vi "Teleop_Calc_Forward.vi"(11 "Teleop Local Data in":T1) -> (3 "Teleop Local Data out":T1)   [LabVIEW 2016]
uses:
  Typedefs/typedef_cluster_Teleop Local Data.ctl
  Typedefs/typedef_enum_Joystick Axes.ctl
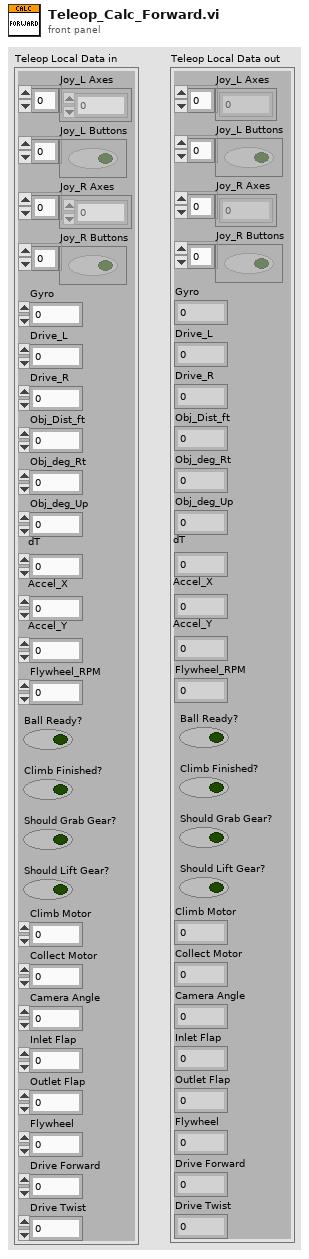
[diagram p1: front panel]
types:
  T1 = typedef "typedef_cluster_Teleop Local Data.ctl" = cluster{"Joy_L Axes":dbl[], "Joy_L Buttons":bool[], "Joy_R Axes":dbl[], "Joy_R Buttons":bool[], "Gyro":dbl, "Drive_L":i32, "Drive_R":i32, "Obj_Dist_ft":dbl, "Obj_deg_Rt":dbl, "Obj_deg_Up":dbl, "dT":dbl, "Accel_X":dbl, "Accel_Y":dbl, "Flywheel_RPM":dbl, "Ball Ready?":bool, "Climb Finished?":bool, "Should Grab Gear?":bool, "Should Lift Gear?":bool, "Climb Motor":dbl, "Collect Motor":dbl, "Camera Angle":dbl, "Inlet Flap":dbl, "Outlet Flap":dbl, "Flywheel":dbl, "Drive Forward":dbl, "Drive Twist":dbl}
  T2 = typedef "typedef_enum_Joystick Axes.ctl" = enum16{"LeftRight", "ForeBack", "Twist", "Throttle"}
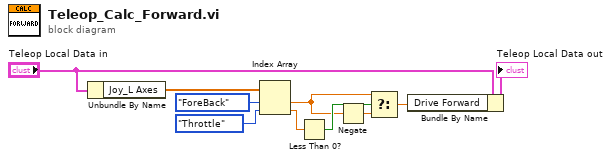
[diagram p0: block diagram]
diagram:
  n1 = Unbundle By Name("Teleop Local Data in") -> ("Joy_L Axes"=w7:dbl[])
  n2 = Index Array(array=w7, index #1=typedef_enum_Joystick_Axes."ForeBack" ("Joystick Axes"), index #2=typedef_enum_Joystick_Axes."Throttle" ("Joystick Axes")) -> (element #1=w1:dbl, element #2=w5:dbl)
  n3 = Less Than 0?(x=w5) -> (x < 0?=w4:bool)
  n4 = Negate(x=w1) -> (-x=w2:dbl)
  n5 = Select(t=w1, s=w4, f=w2) -> (s? t:f=w3:dbl)
  n6 = Bundle By Name(cluster="Teleop Local Data in", "Drive Forward"=w3) -> (→"Teleop Local Data out":T1)
